vi "rqp_Write Termex.vi"(4 "Show in Debugger?":bool=TRUE, 6 "Message Priority":T1=enum."Normal", 7 "Caller in":refnum<class "Worker.lvclass">, 8 "error in":errorcluster, 10 "Data in":T2, 11 "Modbus PLC in":refnum<class "Modbus PLC.lvclass">) -> (0 "error out":errorcluster, 3 "dup Modbus PLC out":refnum<class "Modbus PLC.lvclass">, 5 "dup Caller out":refnum<class "Worker.lvclass">)   [LabVIEW 2023, in "Modbus PLC.lvlib" / "Modbus PLC.lvclass"]
doc: "This VI sends a <b>Public API Request</b> message to an MHL case of the Worker that owns this VI.\n---\nWorkers Public API Request Case"
uses:
  Modbus PLC.lvclass
  C:/Program Files/National Instruments/LabVIEW 2023/vi.lib/addons/_Workers/Library/Classes/Worker/Worker.lvclass
  <vilib>/addons/_Workers/Library/Classes/Worker/Worker.lvclass
  rqp_Write Termex.ctl
  <vilib>/addons/_Workers/Library/Classes/Message/Priority.ctl
  <vilib>/addons/_Workers/Library/Case Label.ctl
  <vilib>/addons/_Workers/Library/Classes/Message Queue/Message Queue.lvclass
  <vilib>/addons/_Workers/Library/Workers.lvlib
  <vilib>/addons/_Workers/Library/Classes/Message/Message.lvclass
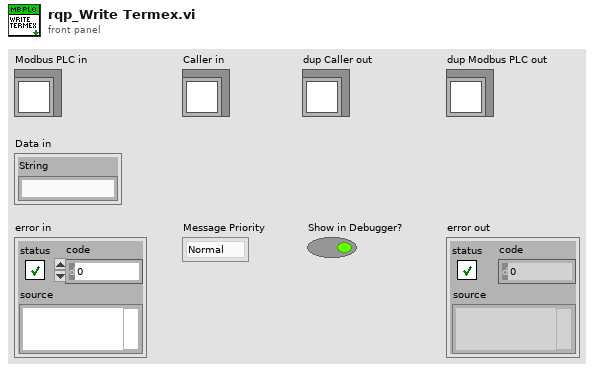
[diagram p1: front panel]
types:
  T1 = typedef "Workers.lvlib/Message.lvclass/Priority.ctl" = enum16{"Low", "Normal", "High"}
  T2 = typedef "Modbus PLC.lvlib/Modbus PLC.lvclass/rqp_Write Termex.ctl" = cluster{"String":string}
  T3 = typedef "Workers.lvlib/Case Label.ctl" = string
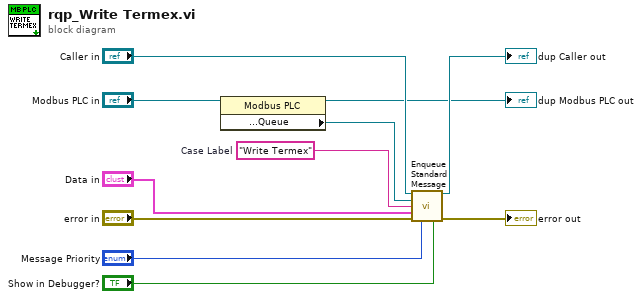
[diagram p0: block diagram]
diagram:
  w1 = T3 "Write Termex"  # Case Label
  n1 = property class="Modbus PLC"(reference="Modbus PLC in") -> (reference out=→"dup Modbus PLC out":refnum<class "Modbus PLC.lvclass">, "Accessors:Read:Public API:Queue"=w2:refnum<class "Message Queue.lvclass">)  [unwired: 1 in, 1 out]
  n2 = call-dynamic "Enqueue Standard Message.vi"("Worker"="Caller in", "Message Queue"=w2, "Case Label"=w1, "Data"="Data in", "error in (no error)"="error in", "Priority (Normal)"="Message Priority", "Send Message to Debugger? (T)"="Show in Debugger?") -> ("dup Worker out"=→"dup Caller out":refnum<class "Worker.lvclass">, "error out"=→"error out":errorcluster)  [unwired: 7 in]
